vi "ParseGenericBooleanExpression.vi"(8 "error in (no error)":errorcluster, 10 "ConditionExpression":string, 11 "bool trigger array":bool[](array[boolean])) -> (0 "error out":errorcluster, 3 "expression":string)   [LabVIEW 2017, in "Trigger.lvlib"]
uses:
  <vilib>/addons/InsightCM/Devices/Shared/Common/Trigger/Trigger.lvlib
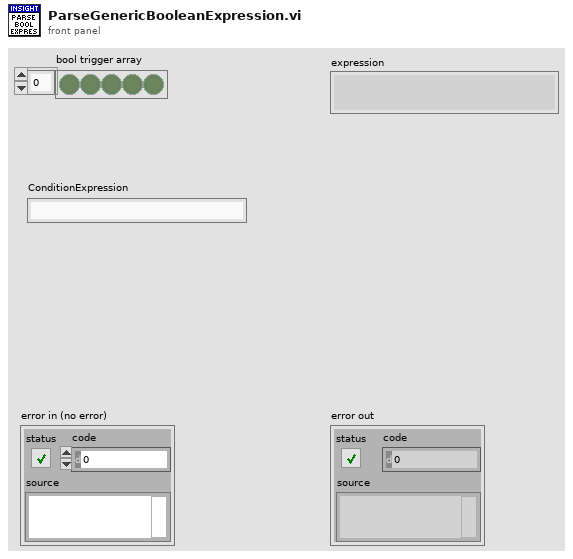
[diagram p1: front panel]
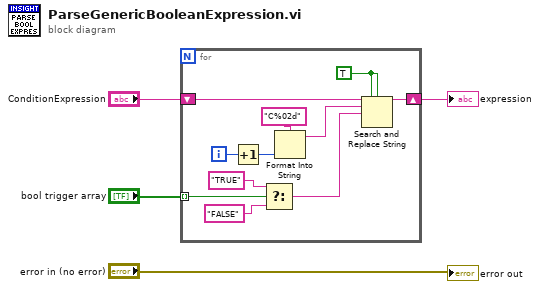
[diagram p0: block diagram]
diagram:
  n1 = for {
    shift-right: [w10] -> w1
    shift-left: "ConditionExpression" -> [w11]
    tunnel: "bool trigger array" -> [w12] mode=indexing
    i -> [w14]
    w9 = TRUE ("replace all? (F)")
    n2 = Increment(x=w14) -> (x+1=w13:i32)
    n3 = Select(t="TRUE" ("format string"), s=w12, f="FALSE" ("format string")) -> (s? t:f=w5:string)
    n4 = Format Into String(format string="C%02d", w13) -> (resulting string=w8:string)  [unwired: 2 in, 1 out]
    n5 = Search and Replace String(replace all?=w9, case sensitive?=w9, input string=w11, search string=w8, replace string=w5) -> (result string=w10:string)  [unwired: 3 in, 3 out]
  }
  "expression" <- w1
  "error out" <- "error in (no error)"
